vi "Download and Upload File.vi"   [LabVIEW 2018]
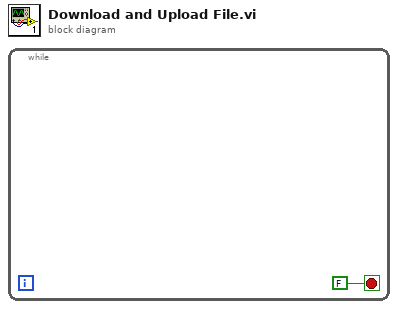
[diagram p0: block diagram]
diagram:
  n1 = while {
    stop <- FALSE stop-if-true
  }
